vi "UTIL_Parse_Vector_File.vi"(11 "data":dbl[](array[numeric])) -> (0 "Measure":T1, 1 "Drain!Fill":bool, 2 "Cluster":cluster{dbl, dbl, dbl}, 3 "Array":dbl[](array[numeric]))   [LabVIEW 2024]
uses:
  Control Definitions/Def Measure.ctl
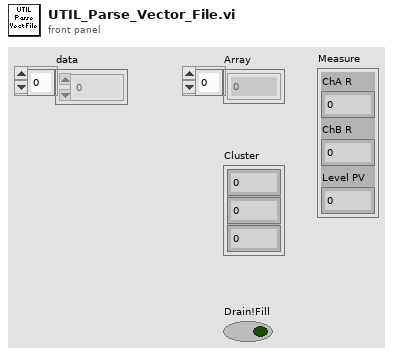
[diagram p1: front panel]
types:
  T1 = typedef "Def Measure.ctl" = cluster{"ChA R":dbl, "ChB R":dbl, "Level PV":dbl}
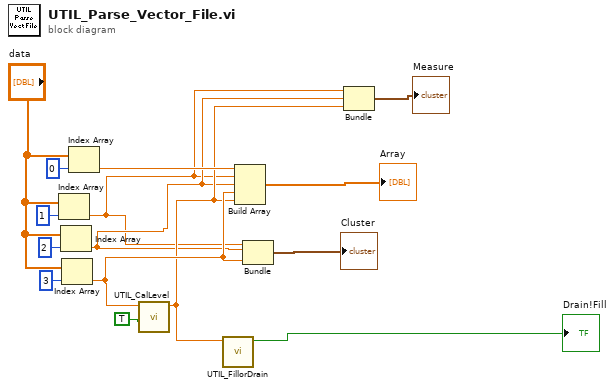
[diagram p0: block diagram]
diagram:
  n1 = Index Array(array="data", index=1) -> (element=w1:dbl)
  n2 = Index Array(array="data", index=2) -> (element=w3:dbl)
  n3 = Index Array(array="data", index=3) -> (element=w13:dbl)
  n4 = Index Array(array="data", index=0) -> (element=w12:dbl)
  n5 = call "UTIL_CalLevel.vi"("Key is In?"=TRUE, "Input"=w13) -> ("PVs"=w4:dbl)  [unwired: 8 in, 1 out]
  n6 = call "UTIL_FillorDrain.vi"("PVs"=w4) -> ("Boolean"=→"Drain!Fill":bool)  [unwired: 10 in]
  n7 = Build Array(w12, w1, w3, w13, w4) -> (→"Array":dbl[])
  n8 = Bundle(w1, w3, w13) -> (→"Cluster":cluster{dbl, dbl, dbl})  [unwired: 1 in]
  n9 = Bundle(w1, w3, "PVs"=w4) -> (→"Measure":cluster{dbl, dbl, "PVs":dbl})  [unwired: 1 in]
